vi "AndorImage.vi"() -> ()   [LabVIEW 2014]
panel:
  out "AndorImage":i32[][](array[numeric])
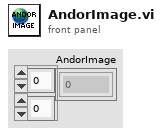
[diagram p1: front panel]
diagram:
